vi "Move padle(SubVI).vi"(8 "Lewy":bool, 9 "Prawy":bool, 10 "Max długości pola paletki":i32, 11 "Obecna pozycja paletki":i32) -> (3 "Nowa pozycja paletki":i32)   [LabVIEW 2018]
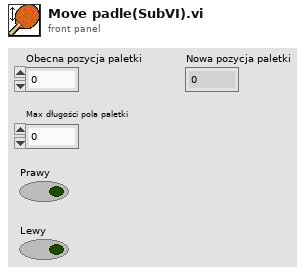
[diagram p1: front panel]
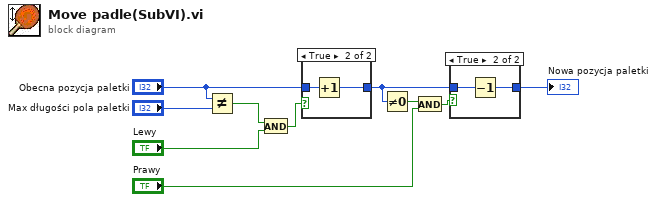
[diagram p0: block diagram]
diagram:
  n1 = Not Equal?(x="Obecna pozycja paletki", y="Max długości pola paletki") -> (x != y?=w8:bool)
  n2 = And(x=w8, y="Lewy") -> (x .and. y?=w9:bool)
  n3 = case shown="True" w9 {
    tunnel: "Obecna pozycja paletki" -> [w11 w13]
    tunnel: [w11 w12] -> w6
    frame False {
    }
    frame True {
      n4 = Increment(x=w13) -> (x+1=w12:i32)
    }
  }
  n5 = Not Equal To 0?(x=w6) -> (x != 0?=w5:bool)
  n6 = And(x=w5, y="Prawy") -> (x .and. y?=w4:bool)
  n7 = case shown="True" w4 {
    tunnel: w6 -> [w14 w16]
    tunnel: [w14 w15] -> w3
    frame False {
    }
    frame True {
      n8 = Decrement(x=w16) -> (x-1=w15:i32)
    }
  }
  "Nowa pozycja paletki" <- w3
